vi "Curtin1_SelectTemplate.vi"(11 "Settings in":T1={"Name of test"="", "Date"=timestamp(0 s since 1904-01-01), "Location"="", "Template"="", "Soundcard"="", "resolution"=32, "Sampling rate"=48000, "Ch1 Gain "=25.0, "Ch2 Gain"=10.0, "Sample time (s)"=0.3, "Pre-trigger (s)"=0.01, "Hammer Threshold"=10.0, "Positions"=12, "Taps/Position"=5, "Set Names"="", "Freq resolution"=10.0, "Hammer cutoff"=0.0, "Mic cutoff"=0.0, "Double bounce "=0.0, "Hammer Cal"=10.0, "dB Offset"=0.0, "Accel Cal"=10.0, "Vibrometer Cal"=0.0, "Mic Cal"=0.0, "Output"=2, "Voltage Cal"=0.01, "Vibrometer Port"="ASRL27::INSTR", "Range"=4, "High Pass"=2, "Bandwidth"=4, "X Range"=[], "Y Range"=[], "dB Spread"=0.0, "Trigger"=0, "Ch_1"=25, "Ch_2"=25, "flip?"=FALSE, "60Hz"=FALSE, "Time offset"=0.0, "Piezo Cal"=1.0, "Default Notes"=""} {"Ch_2" min=1 step=1; "Ch_1" min=1 max=100 step=1; "Trigger" items=["Hammer (force)", "Self-tap", "Spacebar"]; "Bandwidth" items=["1 kHz"=1, "5 kHz"=5, "10 kHz"=10, "25 kHz"=25, "50 kHz"=50, "100 kHz"=100]; "High Pass" items=["Off", "13 Hz", "104 Hz"]; "Range" items=["10 mm/s"=1, "20 mm/s"=2, "50 mm/s"=5, "100 mm/s"=10, "200 mm/s"=20, "500 mm/s"=50, "1 m/s"=100, "2 m/s"=200]; "Output" items=["Accelerometer", "Speed (from acceleration)", "Microphone", "Vibrometer", "Piezo"]; "Voltage Cal" format="%#_13g"; "Ch2 Gain" format="%#_13g"; "Ch1 Gain" format="%#_13g"; "Double bounce" min=0.0; "Mic cutoff" min=0.0 format="%#_4g"; "Hammer cutoff" min=0.0 format="%#_4g"; "Freq resolution" min=0.0; "Pre-trigger (s)" format="%#_13g"; "Date" format="%<%H:%M\n%d/%m/%y>T"; "resolution" items=["16 bit"=16, "24 bit"=24, "32 bit"=32]; "Sampling rate" items=["22050 samp/s"=22050, "44100 samp/s"=44100, "48000 samp/s"=48000]}) -> (1 "New Template":string, 3 "Settings out":T1={"Name of test"="", "Date"=timestamp(0 s since 1904-01-01), "Location"="", "Template"="", "Soundcard"="", "resolution"=32, "Sampling rate"=48000, "Ch1 Gain "=25.0, "Ch2 Gain"=10.0, "Sample time (s)"=0.3, "Pre-trigger (s)"=0.01, "Hammer Threshold"=10.0, "Positions"=12, "Taps/Position"=5, "Set Names"="", "Freq resolution"=10.0, "Hammer cutoff"=0.0, "Mic cutoff"=0.0, "Double bounce "=0.0, "Hammer Cal"=10.0, "dB Offset"=0.0, "Accel Cal"=10.0, "Vibrometer Cal"=0.0, "Mic Cal"=0.0, "Output"=2, "Voltage Cal"=0.01, "Vibrometer Port"="ASRL27::INSTR", "Range"=4, "High Pass"=2, "Bandwidth"=4, "X Range"=[], "Y Range"=[], "dB Spread"=0.0, "Trigger"=0, "Ch_1"=25, "Ch_2"=25, "flip?"=FALSE, "60Hz"=FALSE, "Time offset"=0.0, "Piezo Cal"=1.0, "Default Notes"=""} {"Ch_2" min=1 step=1; "Ch_1" min=1 max=100 step=1; "Trigger" items=["Hammer (force)", "Self-tap", "Spacebar"]; "Bandwidth" items=["1 kHz"=1, "5 kHz"=5, "10 kHz"=10, "25 kHz"=25, "50 kHz"=50, "100 kHz"=100]; "High Pass" items=["Off", "13 Hz", "104 Hz"]; "Range" items=["10 mm/s"=1, "20 mm/s"=2, "50 mm/s"=5, "100 mm/s"=10, "200 mm/s"=20, "500 mm/s"=50, "1 m/s"=100, "2 m/s"=200]; "Output" items=["Accelerometer", "Speed (from acceleration)", "Microphone", "Vibrometer", "Piezo"]; "Voltage Cal" format="%#_13g"; "Ch2 Gain" format="%#_13g"; "Ch1 Gain" format="%#_13g"; "Double bounce" min=0.0; "Mic cutoff" min=0.0 format="%#_4g"; "Hammer cutoff" min=0.0 format="%#_4g"; "Freq resolution" min=0.0; "Pre-trigger (s)" format="%#_13g"; "Date" format="%<%H:%M\n%d/%m/%y>T"; "resolution" items=["16 bit"=16, "24 bit"=24, "32 bit"=32]; "Sampling rate" items=["22050 samp/s"=22050, "44100 samp/s"=44100, "48000 samp/s"=48000]})   [LabVIEW 2022 SP3]
uses:
  PreferencesControl.ctl
panel:
  in  "Settings File":bool
  in  "delete":bool
  in  "Cancel Button":bool
  in  "OK Button":bool
  in  "Template File":string(combo)
  in  "Edit":bool
  # "Hz"
  # "dB"
  # "dB"
  # "sec"
  # "sec"
  # "mV/Pa"
  # "mV/m/s2"
  # "mV/mm/s"
  # "V/N"
  # "sec"
  # "sec"
  # "mV/N"
  # "a.u."
  # "a.u."
  # "sec"
  # "Hz"
  # "dB"
  # "dB"
  # "sec"
  # "sec"
  # "mV/Pa"
  # "mV/m/s2"
  # "mV/mm/s"
  # "V/N"
  # "sec"
  # "sec"
  # "mV/N"
  # "a.u."
  # "a.u."
  # "sec"
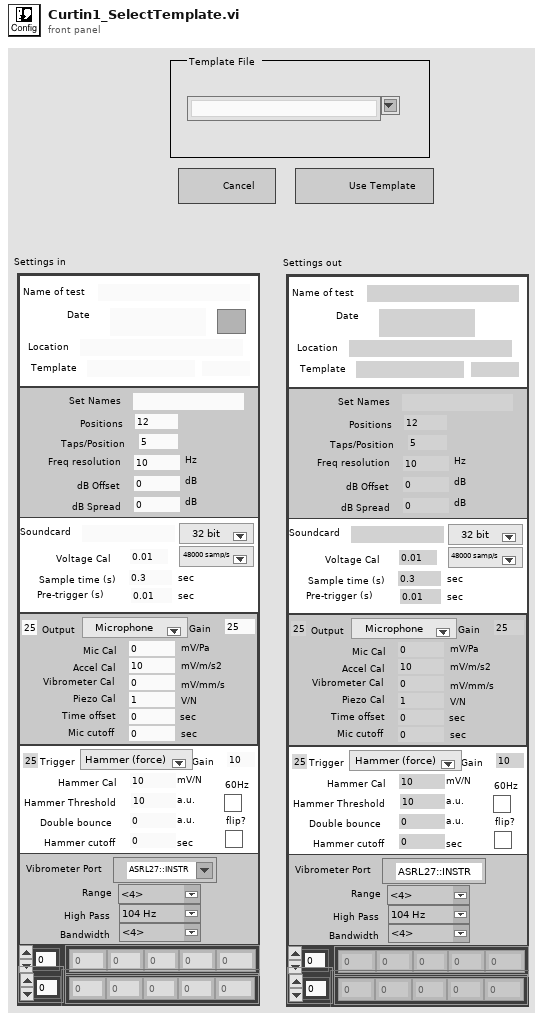
[diagram p1: front panel]
types:
  T1 = typedef "PreferencesControl.ctl" = cluster{"Name of test":string, "Date":timestamp, "Location":string, "Template":string, "Soundcard":string, "resolution":u16, "Sampling rate":u16, "Ch1 Gain ":dbl, "Ch2 Gain":dbl, "Sample time (s)":dbl, "Pre-trigger (s)":dbl, "Hammer Threshold":dbl, "Positions":i16, "Taps/Position":i16, "Set Names":string, "Freq resolution":dbl, "Hammer cutoff":dbl, "Mic cutoff":dbl, "Double bounce ":dbl, "Hammer Cal":dbl, "dB Offset":dbl, "Accel Cal":dbl, "Vibrometer Cal":dbl, "Mic Cal":dbl, "Output":u16, "Voltage Cal":dbl, "Vibrometer Port":refnum<visa-resource-name>, "Range":u16, "High Pass":u16, "Bandwidth":u16, "X Range":cluster{"Minimum":dbl, "Maximum":dbl, "Increment":dbl, "Minor Increment":dbl, "Start":dbl}[], "Y Range":cluster{"Minimum":dbl, "Maximum":dbl, "Increment":dbl, "Minor Increment":dbl, "Start":dbl}[], "dB Spread":dbl, "Trigger":u16, "Ch_1":u8, "Ch_2":u8, "flip?":bool, "60Hz":bool, "Time offset":dbl, "Piezo Cal":dbl, "Default Notes":string}
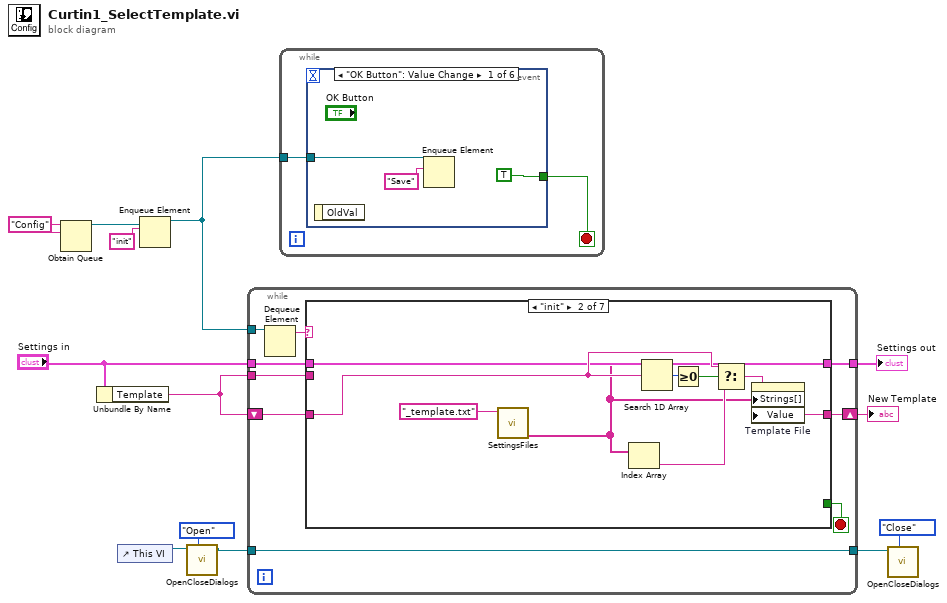
[diagram p0: block diagram]
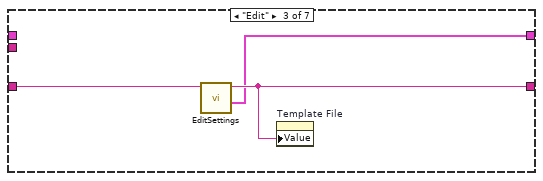
[diagram p3: hidden frame]
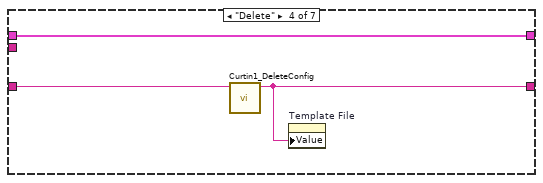
[diagram p4: hidden frame]
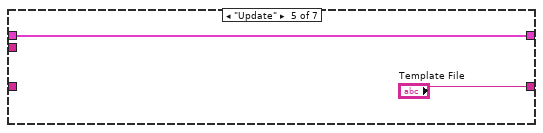
[diagram p5: hidden frame]
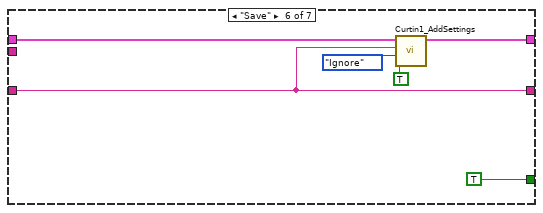
[diagram p6: hidden frame]
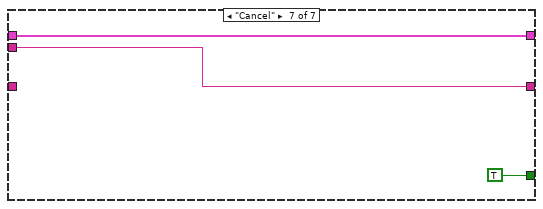
[diagram p7: hidden frame]
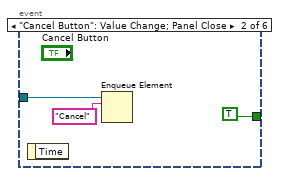
[diagram p8: hidden frame]
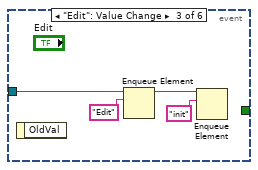
[diagram p9: hidden frame]
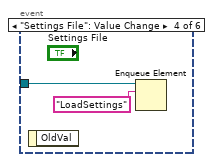
[diagram p10: hidden frame]
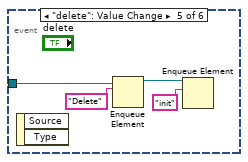
[diagram p11: hidden frame]
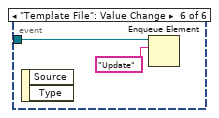
[diagram p12: hidden frame]
diagram:
  w13 = "Config" ("name (unnamed)")
  n1 = Obtain Queue(name (unnamed)=w13, element data type=w13) -> (queue out=w12:refnum<queue>)  [unwired: 3 in, 2 out]
  n2 = Unbundle By Name("Settings in") -> ("Template"=w10:string)
  n3 = control-ref of="This VI"() -> (w4:refnum<vi>)
  n4 = Enqueue Element(queue=w12, element="init") -> (queue out=w9:refnum<queue>)  [unwired: 2 in, 2 out]
  n5 = call "OpenCloseDialogs.vi"("Task"=enum16{"Open", "Close"}."Open", "VI in"=w4) -> ("VI out"=w1:refnum<vi>)  [unwired: 8 in, 1 out]
  n6 = while {
    tunnel: w9 -> [w21]
    tunnel: w10 -> [w20]
    shift-right: [w15] -> w6
    shift-left: w10 -> [w19]
    tunnel: "Settings in" -> [w17]
    tunnel: [w16] -> w7
    tunnel: [w14] -> w2
    tunnel: w1 -> [w14]
    stop <- w18 stop-if-true
    n7 = Dequeue Element(queue=w21) -> (element=w22:string)  [unwired: 2 in, 3 out]
    n8 = case shown="\"init\"" w22 {
      tunnel: w20 -> [_ _ _ _ _ _ w49]
      tunnel: [w24 w29 w34 w37 "Template File" w43 w49] -> w15
      tunnel: w19 -> [w24 w28 w35 w38 _ w43 _]
      tunnel: [_ _ _ _ _ TRUE TRUE] -> w18
      tunnel: w17 -> [w23 w27 _ w36 w39 w45 w47]
      tunnel: [w23 w27 w33 w36 w39 w44 w47] -> w16
      frame Default {
      }
      frame "init" {
        n9 = call "SettingsFiles.vi"("settings file name"="_template.txt" ("pattern")) -> ("filenames"=w25:string[])  [unwired: 9 in, 1 out]
        n10 = Index Array(array=w25) -> (element=w32:string)  [unwired: 1 in]
        n11 = Search 1D Array(1D array=w25, element=w28) -> (index of element=w30:i32)  [unwired: 1 in]
        n12 = Greater Or Equal To 0?(x=w30) -> (x >= 0?=w31:bool)
        n13 = Select(t=w28, s=w31, f=w32) -> (s? t:f=w29:string)
        n14 = property on="Template File" class="CmbBox"("Strings[]"=w25, "Value"=w29) -> ()  [unwired: 2 in, 2 out]
      }
      frame "Edit" {
        n15 = call "EditSettings.vi"("Template in"=w35) -> ("Settings out"=w33:T1, "Template out"=w34:string)  [unwired: 9 in]
        n16 = property on="Template File" class="CmbBox"("Value"=w34) -> ()  [unwired: 2 in, 2 out]
      }
      frame "Delete" {
        n17 = call "Curtin1_DeleteConfig.vi"("Test Configuration"=w38) -> ("New File"=w37:string)  [unwired: 10 in]
        n18 = property on="Template File" class="CmbBox"("Value"=w37) -> ()  [unwired: 2 in, 2 out]
      }
      frame "Update" {
      }
      frame "Save" {
        n19 = call "Curtin1_AddSettings.vi"("Date?"=TRUE, "Check?"=enum16{"Ignore", "Check", "Replace"}."Ignore", "Template"=w43, "Settings in"=w45) -> ("Settings Out"=w44:T1)  [unwired: 6 in, 1 out]
      }
      frame "Cancel" {
      }
    }
  }
  "Settings out" <- w7
  "New Template" <- w6
  n20 = while {
    tunnel: w9 -> [w50]
    stop <- w51 stop-if-true
    n21 = event shown="[0] \"OK Button\": Value Change" {
      selector: _ -> [_ _ _ _ _ _]
      dyn-events: _ -> [_ _ _ _ _ _]
      timeout: _ -> [_ _ _ _ _ _]
      tunnel: [TRUE ("OK Button") TRUE ("OK Button") _ _ _ _] -> w51
      tunnel: w50 -> [w52 w55 w60 w62 w66 w68]
      event "OK Button": Value Change {
        n22 = event-data() -> ()  [unwired: 1 in, 1 out]
        n23 = Enqueue Element(queue=w52, element="Save") -> ()  [unwired: 2 in, 3 out]
      }
      event "Cancel Button": Value Change; Panel Close {
        n24 = event-data() -> ()  [unwired: 1 in, 1 out]
        n25 = Enqueue Element(queue=w55, element="Cancel") -> ()  [unwired: 2 in, 3 out]
      }
      event "Edit": Value Change {
        n26 = event-data() -> ()  [unwired: 1 in, 1 out]
        n27 = Enqueue Element(queue=w60, element="Edit") -> (queue out=w58:refnum<queue>)  [unwired: 2 in, 2 out]
        n28 = Enqueue Element(queue=w58, element="init") -> ()  [unwired: 2 in, 3 out]
      }
      event "Settings File": Value Change {
        n29 = event-data() -> ()  [unwired: 1 in, 1 out]
        n30 = Enqueue Element(queue=w62, element="LoadSettings") -> ()  [unwired: 2 in, 3 out]
      }
      event "delete": Value Change {
        n31 = event-data() -> ()  [unwired: 1 in, 2 out]
        n32 = Enqueue Element(queue=w66, element="Delete") -> (queue out=w64:refnum<queue>)  [unwired: 2 in, 2 out]
        n33 = Enqueue Element(queue=w64, element="init") -> ()  [unwired: 2 in, 3 out]
      }
      event "Template File": Value Change {
        n34 = event-data() -> ()  [unwired: 1 in, 2 out]
        n35 = Enqueue Element(queue=w68, element="Update") -> ()  [unwired: 2 in, 3 out]
      }
    }
  }
  n36 = call "OpenCloseDialogs.vi"("Task"=enum16{"Open", "Close"}."Close", "VI in"=w2) -> ()  [unwired: 8 in, 2 out]
